vi "confirm_popup.vi"(5 "Warning(T)/Inf(F)":bool, 7 "Title":string, 8 "error_in":errorcluster, 9 "False Label":string, 10 "True Label":string, 11 "Message":string) -> (0 "error_out":errorcluster, 3 "Result":bool)   [LabVIEW 2020]
uses:
  AULocalize/SubVIs/Get Localized Phrase Compact Interface 0D.vi
panel:
  out "Project Title 2":string
  out "Message copy":string
  in  "False":bool
  in  "True":bool
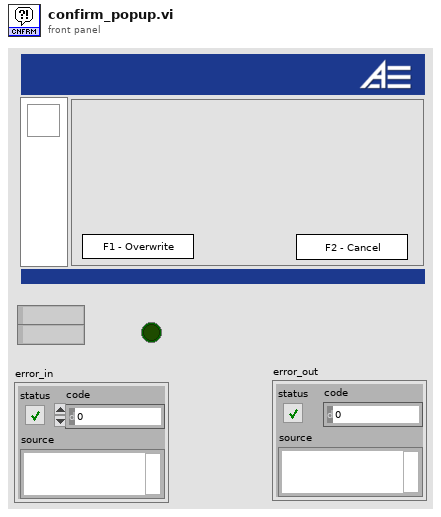
[diagram p1: front panel]
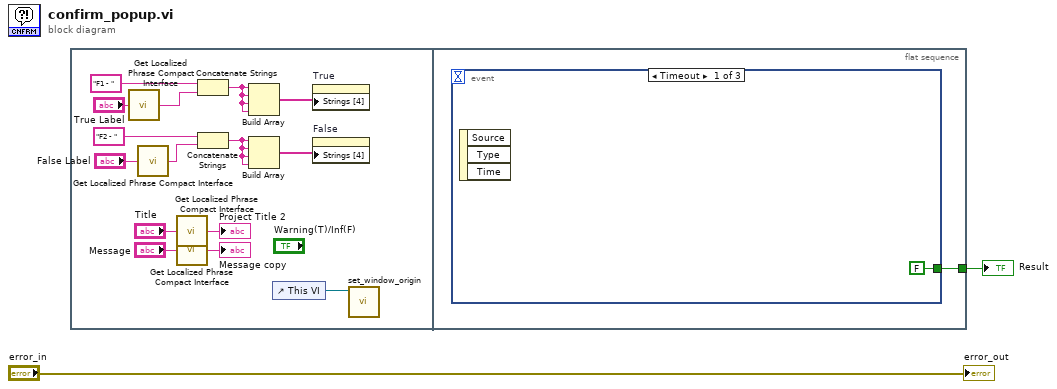
[diagram p0: block diagram]
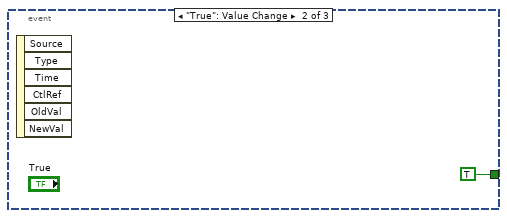
[diagram p2: hidden frame]
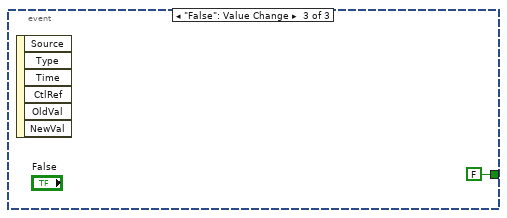
[diagram p3: hidden frame]
diagram:
  n1 = flat-sequence {
    tunnel: [w18] -> w2
    frame #0 {
      n2 = call-poly "Get Localized Phrase Compact Interface.vi"("Key"="True Label") -> ("Translated Phrase"=w5:string)
      n3 = call-poly "Get Localized Phrase Compact Interface.vi"("Key"="False Label") -> ("Translated Phrase"=w6:string)
      n4 = call-poly "Get Localized Phrase Compact Interface.vi"("Key"="Title") -> ("Translated Phrase"=→"Project Title 2":string)
      n5 = call-poly "Get Localized Phrase Compact Interface.vi"("Key"="Message") -> ("Translated Phrase"=→"Message copy":string)
      n6 = Concatenate Strings("F1 - ", w5) -> (w9:string)
      n7 = Concatenate Strings("F2 - ", w6) -> (w8:string)
      n8 = Build Array(w9, w9, w9, w9) -> (w13:string[])
      n9 = Build Array(w8, w8, w8, w8) -> (w12:string[])
      n10 = control-ref of="This VI"() -> (w7:refnum<vi>)
      n11 = property on="True" class="Bool"("Strings [4]"=w13) -> ()  [unwired: 2 in, 2 out]
      n12 = property on="False" class="Bool"("Strings [4]"=w12) -> ()  [unwired: 2 in, 2 out]
      n13 = call "set_window_origin.vi"("this_vi_reference"=w7) -> ()  [unwired: 10 in, 1 out]
    }
    frame #1 {
      n14 = event shown="[0] Timeout" {
        selector: _ -> [_ _ _]
        dyn-events: _ -> [_ _ _]
        timeout: _ -> [_ _ _]
        tunnel: [FALSE TRUE FALSE] -> w18
        event Timeout {
          n15 = event-data() -> ()  [unwired: 1 in, 3 out]
        }
        event "True": Value Change {
          n16 = event-data() -> ()  [unwired: 1 in, 6 out]
        }
        event "False": Value Change {
          n17 = event-data() -> ()  [unwired: 1 in, 6 out]
        }
      }
    }
  }
  "Result" <- w2
  "error_out" <- "error_in"
